vi "Lookup Node by ID.vi"(8 "error in (no error)":errorcluster, 10 "node_id":u32, 11 "DiscoveryService in":refnum<class "NodeDiscovery.lvclass">) -> (0 "error out":errorcluster, 2 "Node":T1, 3 "DiscoveryService out":refnum<class "NodeDiscovery.lvclass">)   [LabVIEW 2020, in "Vecto.lvlib" / "NodeDiscovery.lvclass"]
uses:
  NodeDiscovery.lvclass
  NodeDiscovery.lvclass/NodeDiscovery.ctl
  proto/ServiceType/Enumeration.ctl
  proto/ServiceType/ServiceType.lvlib
  proto/Service/Data.ctl
  proto/Service/Service.lvlib
  proto/Discovery/Data.ctl
  proto/Discovery/Discovery.lvlib
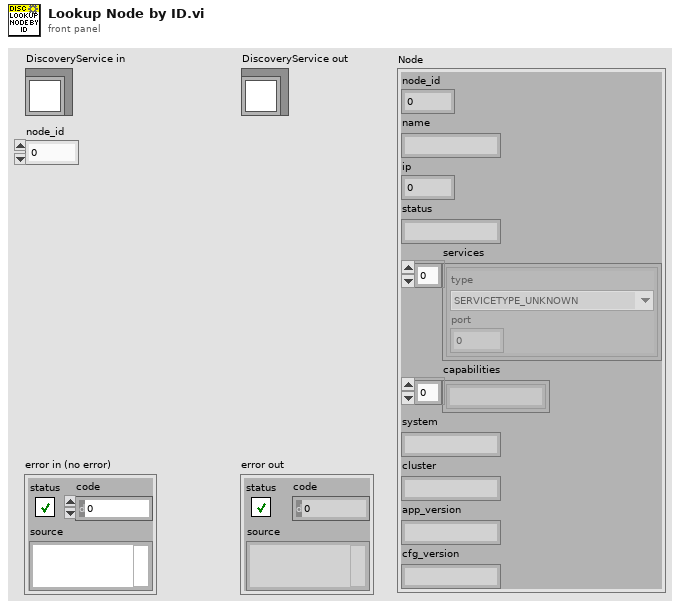
[diagram p1: front panel]
types:
  T1 = typedef "Discovery.lvlib/Data.ctl" = cluster{"node_id":u32, "name":string, "ip":u32, "status":string, "services":T2[], "capabilities":string[], "system":string, "cluster":string, "app_version":string, "cfg_version":string}
  T2 = typedef "Service.lvlib/Data.ctl" = cluster{"type":T3, "port":i32}
  T3 = typedef "ServiceType.lvlib/Enumeration.ctl" = enum16{"SERVICETYPE_UNKNOWN", "SERVICETYPE_TCPSERVER", "SERVICETYPE_HTTPSERVER"}
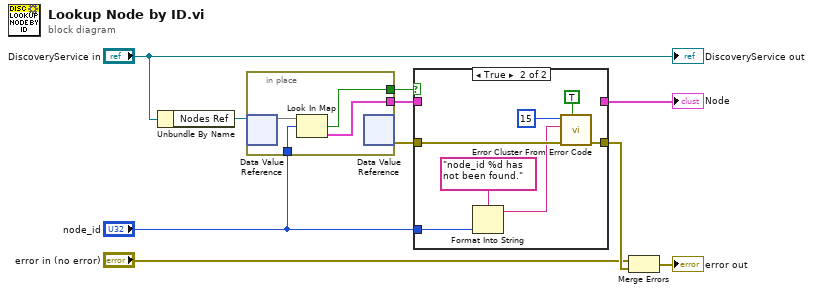
[diagram p0: block diagram]
diagram:
  n1 = Unbundle By Name("DiscoveryService in") -> ("Nodes Ref"=w10:refnum<data-value>)
  n2 = in-place {
    in-place-border: "node_id" -> [w13]
    in-place-border: [w12] -> w8
    in-place-border: [w11] -> w7
    n3 = in-place-dvr #1(w10) -> (w14:map{u32, T1})  [unwired: 1 out]
    n4 = Look In Map(map=w14, key=w13) -> (key not found?=w12:bool, value=w11:T1)  [unwired: 1 in]
    n5 = in-place-dvr #1() -> (w6:errorcluster)  [unwired: 1 in, 1 out]
  }
  n6 = case shown="True" w8 {
    tunnel: w7 -> [w15 _]
    tunnel: w6 -> [_ w22]
    tunnel: [w15 _] -> w5
    tunnel: "node_id" -> [_ w19]
    tunnel: [_ w16] -> w3
    frame False {
    }
    frame True {
      n7 = Format Into String(format string="node_id %d has not been found.", w19) -> (resulting string=w17:string)  [unwired: 2 in, 1 out]
      n8 = call <vilib>:"Error Cluster From Error Code.vi"("show call chain? (False)"=TRUE, "error in (no error)"=w22, "error message (\"\")"=w17, "error code (0)"=15) -> ("error out"=w16:errorcluster)  [unwired: 5 in]
    }
  }
  "Node" <- w5
  n9 = Merge Errors("error in (no error)", w3) -> (→"error out":errorcluster)
  "DiscoveryService out" <- "DiscoveryService in"
